vi "Read Interface Configs.vi"(8 "error in (no error)":errorcluster, 10 "Device Ref in":T1 format="%.0x", 11 "Refnum in":T2) -> (0 "error out":errorcluster, 2 "Item Ref out":T1 format="%.0x", 3 "Refnum out":T2)   [LabVIEW 2015, in "Modbus Master System Explorer.lvlib"]
uses:
  Modbus Master System Explorer.lvlib
  <vilib>/NI Veristand/Custom Device API/Custom Device Item Ref.ctl
  <vilib>/Utility/config.llb/Config Data RefNum.ctl
  Shared/Controls/Interface Type.ctl
  Shared/Constants.vi
  <vilib>/Utility/config.llb/Read Key (String).vi
  <vilib>/Utility/config.llb/Read Key (U32).vi
  <vilib>/NI Veristand/Custom Device API/Set Item Property (U16).vi
  <vilib>/Utility/config.llb/NI_LVConfig.lvlib
  <vilib>/NI VeriStand/Custom Device API/Custom Device API.lvlib
  Shared/Modbus Master Shared.lvlib
  <vilib>/NI VeriStand/Custom Device Tools/Custom Device Utility Library/Custom Device Utility Library.lvlib
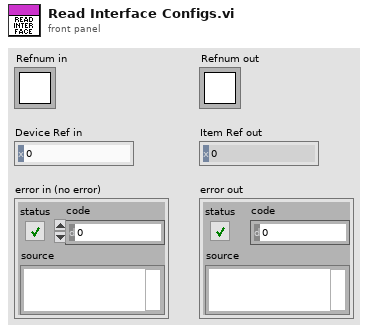
[diagram p1: front panel]
types:
  T1 = typedef "Custom Device API.lvlib/Custom Device Item Ref.ctl" = u64
  T2 = typedef "NI_LVConfig.lvlib/Config Data RefNum.ctl" = refnum<k1>
  T3 = typedef "Modbus Master Shared.lvlib/Interface Type.ctl" = enum16{"TCP Master", "Serial Master", "TCP Slave", "Serial Slave"}
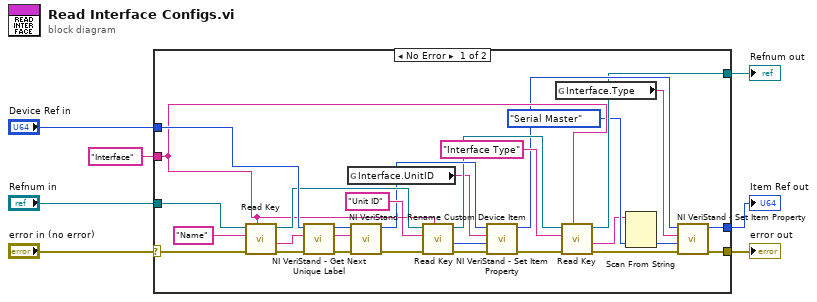
[diagram p0: block diagram]
diagram:
  n1 = case shown="No Error" "error in (no error)" {
    selector: "error in (no error)" -> [w28 w38]
    tunnel: "Device Ref in" -> [w31 w37]
    tunnel: "Refnum in" -> [w30 w39]
    tunnel: "Interface" ("section") -> [w18 _]
    tunnel: [w13 w39] -> w3
    tunnel: [w12 w38] -> w2
    tunnel: [w8 w37] -> w1
    frame No Error {
      n2 = call-poly <vilib>:"Read Key.vi"("section"=w18, "error in (no error)"=w28, "key"="Name", "refnum"=w30) -> ("error out"=w35:errorcluster, "value"=w34:string, "refnum out"=w26:T2)  [unwired: 4 in, 1 out]
      n3 = call <vilib>:"NI VeriStand - Get Next Unique Label.vi"("error in (no error)"=w35, "Label"=w34, "Parent Ref in"=w31) -> ("error out"=w36:errorcluster, "Label out"=w33:string, "Parent Ref dup"=w32:T1)  [unwired: 5 in, 1 out]
      n4 = global read "Constants.vi" "Interface.UnitID"() -> (w17:string)
      n5 = call <vilib>:"NI VeriStand - Rename Custom Device Item.vi"("error in (no error)"=w36, "New Name"=w33, "Item Ref in"=w32) -> ("error out"=w27:errorcluster, "Item Ref out"=w23:T1)  [unwired: 6 in, 1 out]
      n6 = call-poly <vilib>:"Read Key.vi"("section"=w18, "error in (no error)"=w27, "key"="Unit ID", "refnum"=w26) -> ("error out"=w24:errorcluster, "value"=w22:u32, "refnum out"=w20:T2)  [unwired: 4 in, 1 out]
      n7 = call-poly <vilib>:"NI VeriStand - Set Item Property.vi"("error in (no error)"=w24, "Value"=w22, "Property Name"=w17, "Item Ref in"=w23) -> ("error out"=w19:errorcluster, "Item Ref out"=w16:T1)  [unwired: 5 in, 1 out]
      n8 = global read "Constants.vi" "Interface.Type"() -> (w15:string)
      n9 = call-poly <vilib>:"Read Key.vi"("section"=w18, "error in (no error)"=w19, "key"="Interface Type", "refnum"=w20) -> ("error out"=w14:errorcluster, "value"=w10:string, "refnum out"=w13:T2)  [unwired: 4 in, 1 out]
      n10 = Scan From String(input string=w10, default 1=Interface_Type."Serial Master" ("Interface Type")) -> (output 1=w9:T3)  [unwired: 3 in, 3 out]
      n11 = call-poly <vilib>:"NI VeriStand - Set Item Property.vi"("error in (no error)"=w14, "Value"=w9, "Property Name"=w15, "Item Ref in"=w16) -> ("error out"=w12:errorcluster, "Item Ref out"=w8:T1)  [unwired: 5 in, 1 out]
    }
    frame Error {
    }
  }
  "Refnum out" <- w3
  "error out" <- w2
  "Item Ref out" <- w1
